vi "sub vi - Scan Bead.vi"() -> ()   [LabVIEW 2010]
panel:
  in  "Filename":string="test"
  in  "Z step size":dbl=0.2 format="%0.2p"
  in  "Z finish":dbl=7.0 format="%0.2p"
  in  "Z start":dbl=5.0 format="%0.2p"
  in  "X start":dbl=5.0 format="%0.2p"
  in  "X finish":dbl=7.0 format="%0.2p"
  in  "X step size":dbl=0.1 format="%0.2p"
  out "?":cluster{"Y":dbl[], "Y":dbl[]}[](graph)
  in  "Amplitude 13":dbl=0.5 caption="Amplitude (um)" format="%0.2p"
  in  "Desired Frequency 6":dbl=0.3 caption="frequency (Hz)" format="%.2f"
  in  "Waveform Type 7":T1(ring) caption="Waveform Type"
  in  "Phase":u16(ring)=1 items=["Start", "Middle", "Right End"]
  out "X Position 3":dbl
  out "Y Position 3":dbl
  out "Z Position   3":dbl
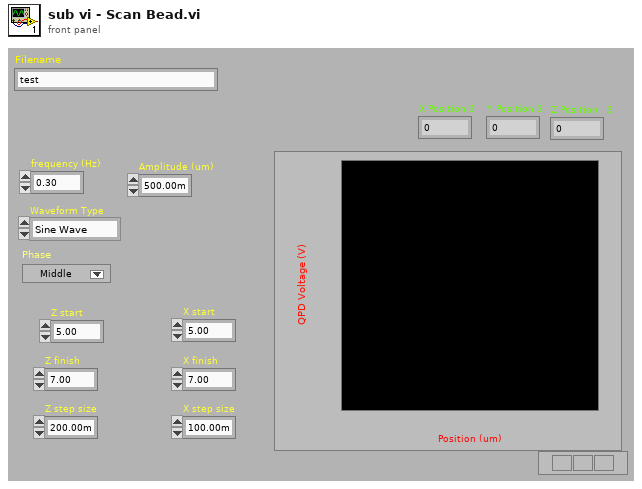
[diagram p1: front panel]
types:
  T1 = enum16{"Sine Wave", "Triangle Wave", "Square Wave", "Sawtooth Wave"}
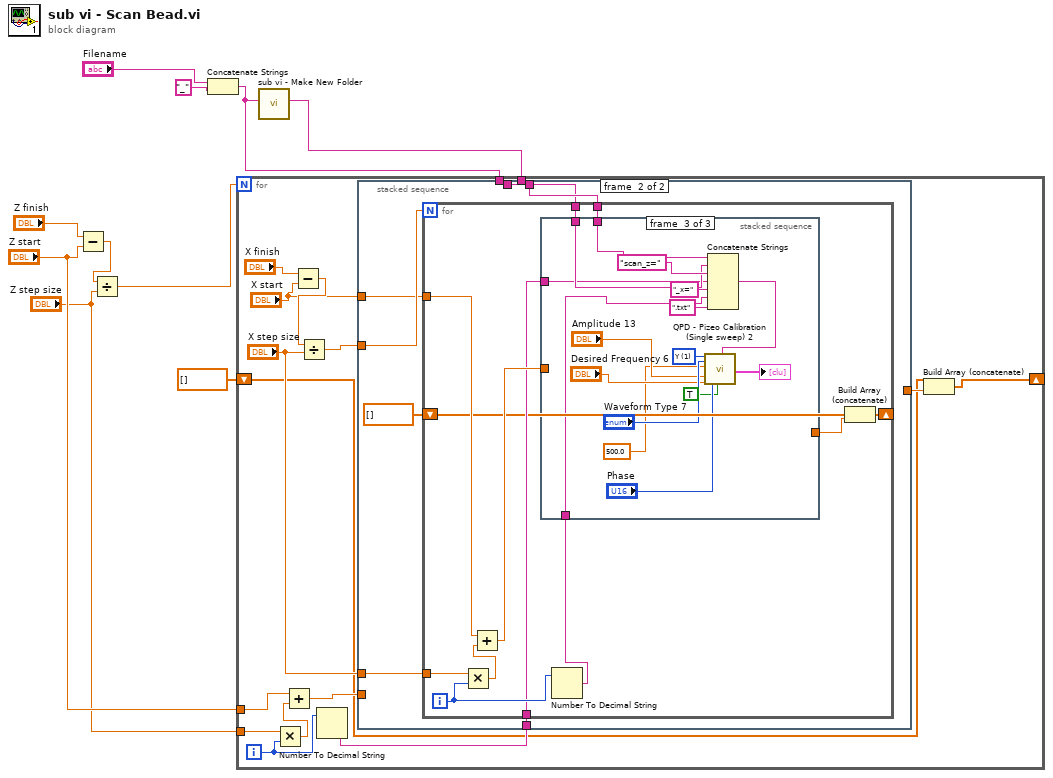
[diagram p0: block diagram]
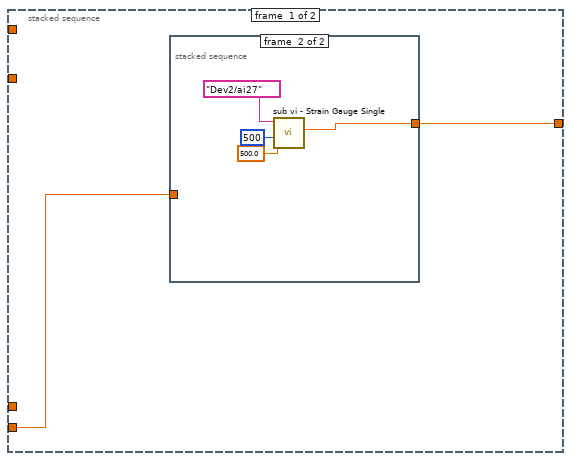
[diagram p2: hidden frame]
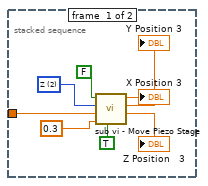
[diagram p3: hidden frame]
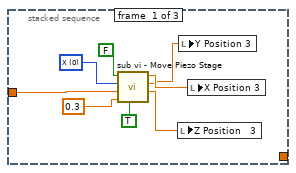
[diagram p4: hidden frame]
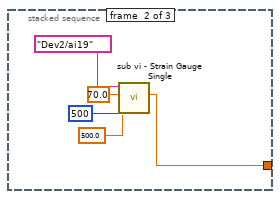
[diagram p5: hidden frame]
diagram:
  n1 = Subtract(x="Z finish", y="Z start") -> (x-y=w10:dbl)
  n2 = Divide(x=w10, y="Z step size") -> (x/y=w8:dbl)
  n3 = Concatenate Strings("Filename", "_" ("string")) -> (w2:string)
  n4 = call "sub vi - Make New Folder.vi"("folder name"=w2) -> ("directory 2"=w3:string)  [unwired: 1 in, 9 out]
  n5 = for {
    N: w8 -> [_]
    tunnel: w3 -> [w26]
    tunnel: w2 -> [w25]
    tunnel: "Z start" -> [w24]
    tunnel: "Z step size" -> [w22]
    shift-right: [w12] -> _
    shift-left: dbl[] [] -> [w11]
    i -> [w15]
    n6 = Multiply(x=w22, y=w15) -> (x*y=w23:dbl)
    n7 = Add(x=w24, y=w23) -> (x+y=w16:dbl)
    n8 = Subtract(x="X finish", y="X start") -> (x-y=w20:dbl)
    n9 = Divide(x=w20, y="X step size") -> (x/y=w19:dbl)
    n10 = Number To Decimal String(number=w15) -> (decimal integer string=w14:string)  [unwired: 1 in]
    n11 = stacked-sequence {
      tunnel: w26 -> [_ w47]
      tunnel: w25 -> [_ w46]
      tunnel: w19 -> [_ w45]
      tunnel: "X start" -> [_ w44]
      tunnel: "X step size" -> [_ w43]
      tunnel: w16 -> [w28 _]
      tunnel: w14 -> [_ w42]
      tunnel: [w27 _] -> w13
      frame #0 {
        n12 = stacked-sequence {
          tunnel: w28 -> [w29 _]
          tunnel: [_ w37] -> w27
          frame #0 {
            w33 = u16 2 items=["X", "Y", "Z"] ("Axis")
            n13 = call "sub vi - Move Piezo Stage.vi"("stop"=TRUE, "Frequency"=0.3 ("frequency"), "Desired Position (um)"=w29, "Axis"=w33, "All Axis"=FALSE) -> ("Z Position"=→"Z Position   3":dbl, "Y Position"=→"Y Position 3":dbl, "X Position"=→"X Position 3":dbl)  [unwired: 4 in]
          }
          frame #1 {
            n14 = call "sub vi - Strain Gauge Single.vi"("rate"=500.0, "# of Samples"=500, "Strain Gauge"=tag "Dev2/ai27") -> ("mean"=w37:dbl)  [unwired: 8 in]
          }
        }
      }
      frame #1 {
        n15 = for {
          N: w45 -> [_]
          tunnel: w47 -> [w59]
          tunnel: w46 -> [w58]
          tunnel: w44 -> [w57]
          tunnel: w43 -> [w56]
          tunnel: w42 -> [w52]
          shift-right: [w50] -> _
          shift-left: dbl[] [] -> [w49]
          i -> [w53]
          n16 = Multiply(x=w56, y=w53) -> (x*y=w55:dbl)
          n17 = Add(x=w57, y=w55) -> (x+y=w54:dbl)
          n18 = Number To Decimal String(number=w53) -> (decimal integer string=w51:string)  [unwired: 1 in]
          n19 = stacked-sequence {
            tunnel: w59 -> [_ _ w81]
            tunnel: w58 -> [_ _ w80]
            tunnel: w54 -> [w63 _ _]
            tunnel: w52 -> [_ _ w77]
            tunnel: w51 -> [_ _ w75]
            tunnel: [_ w71 _] -> w48
            frame #0 {
              w64 = u16 0 items=["X", "Y", "Z"] ("Axis")
              n20 = call "sub vi - Move Piezo Stage.vi"("stop"=TRUE, "Frequency"=0.3 ("frequency"), "Desired Position (um)"=w63, "Axis"=w64, "All Axis"=FALSE) -> ("Z Position"=w60:dbl, "Y Position"=w61:dbl, "X Position"=w62:dbl)  [unwired: 4 in]
              n21 = local write "Z Position   3"(w60) -> ()
              n22 = local write "Y Position 3"(w61) -> ()
              n23 = local write "X Position 3"(w62) -> ()
            }
            frame #1 {
              n24 = call "sub vi - Strain Gauge Single.vi"("rate"=500.0, "# of Samples"=500, "timeout"=70.0, "Strain Gauge"=tag "Dev2/ai19") -> ("mean"=w71:dbl)  [unwired: 7 in]
            }
            frame #2 {
              w73 = u16 1 items=["X", "Y", "Z"] ("Axis")
              n25 = Concatenate Strings(w81, w80, "scan_z=" ("string"), w77, "_x=" ("string"), w75, ".txt" ("string")) -> (w79:string)
              n26 = call "QPD - Pizeo Calibration (Single sweep) 2.vi"("Axis"=w73, "Waveform Type"="Waveform Type 7", "Rate (Hz)"=500.0, "Amplitude"="Amplitude 13", "Desired Frequency"="Desired Frequency 6", "Phase"="Phase", "Save Data"=TRUE, "filename"=w79) -> ("Displacement vs Position 2"=→"?":cluster{dbl[], dbl[]}[])  [unwired: 3 in, 8 out]
            }
          }
          n27 = Build Array (concatenate)(w49, w48) -> (w50:dbl[])
        }
      }
    }
    n28 = Build Array (concatenate)(w11, w13) -> (w12:dbl[])
  }
